vi "Initialize.vi"(8 "error in":errorcluster, 11 "Reversi in":refnum<class "Reversi.lvclass">) -> (0 "error out":errorcluster, 3 "Reversi out":refnum<class "Reversi.lvclass">)   [LabVIEW 2020, in "Reversi.lvlib" / "Reversi.lvclass"]
uses:
  Reversi.lvclass
  Space Ring.ctl
  Space Cluster.ctl
  Space Coordinates.ctl
  Reversi.lvclass/Reversi.ctl
  <vilib>/Utility/error.llb/Clear Errors.vi
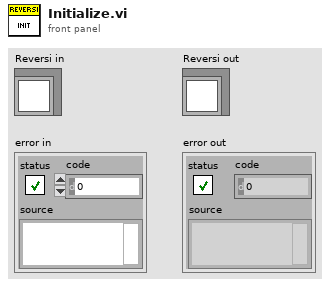
[diagram p1: front panel]
types:
  T1 = typedef "Reversi.lvlib/Reversi.lvclass/Space Cluster.ctl" = cluster{"Coordinates":T2, "Ring":T3}
  T2 = typedef "Reversi.lvlib/Reversi.lvclass/Space Coordinates.ctl" = cluster{"Row":i32, "Column":i32}
  T3 = typedef "Reversi.lvlib/Reversi.lvclass/Space Ring.ctl" = u16
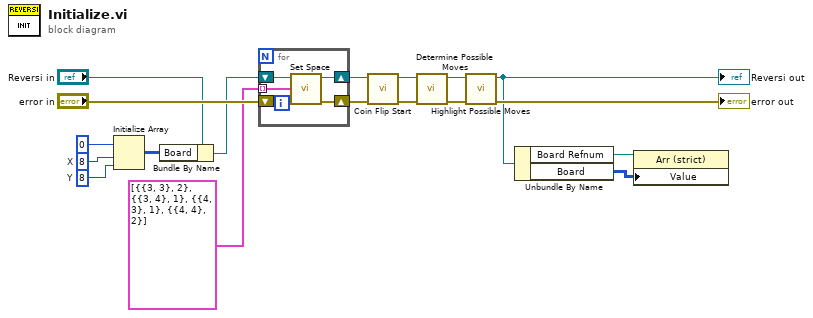
[diagram p0: block diagram]
diagram:
  w14 = 8  # Y
  w15 = 8  # X
  n1 = Initialize Array(T3 0 ("Space Ring"), w15, w14) -> (w9:T3[][])
  n2 = Bundle By Name(cluster="Reversi in", "Board"=w9) -> (w13:refnum<class "Reversi.lvclass">)
  n3 = for {
    shift-right: [w20] -> w6
    shift-left: w13 -> [w21]
    shift-right: [w22] -> w5
    shift-left: "error in" -> [w23]
    tunnel: T1[] [{"Coordinates"={"Row"=3, "Column"=3}, "Ring"=2}, {"Coordinates"={"Row"=3, "Column"=4}, "Ring"=1}, {"Coordinates"={"Row"=4, "Column"=3}, "Ring"=1}, {"Coordinates"={"Row"=4, "Column"=4}, "Ring"=2}] -> [w19] mode=indexing
    n4 = call "Set Space.vi"("error in (no error)"=w23, "Space"=w19, "Reversi in"=w21) -> ("error out"=w22:errorcluster, "Reversi out"=w20:refnum<class "Reversi.lvclass">)  [unwired: 7 in]
  }
  n5 = call "Coin Flip Start.vi"("error in (no error)"=w5, "Reversi in"=w6) -> ("error out"=w18:errorcluster, "Reversi out"=w10:refnum<class "Reversi.lvclass">)  [unwired: 8 in]
  n6 = call "Determine Possible Moves.vi"("error in (no error)"=w18, "Reversi in"=w10) -> ("error out"=w3:errorcluster, "Reversi out"=w4:refnum<class "Reversi.lvclass">)  [unwired: 8 in]
  n7 = call "Highlight Possible Moves.vi"("error in (no error)"=w3, "Reversi in"=w4) -> ("error out"=→"error out":errorcluster, "Reversi out"=w1:refnum<class "Reversi.lvclass">)  [unwired: 8 in]
  "Reversi out" <- w1
  n8 = Unbundle By Name(w1) -> ("Board Refnum"=w7:refnum<vi>, "Board"=w8:T3[][])
  n9 = property class="Arr (strict)"(reference=w7, "Value"=w8) -> ()  [unwired: 1 in, 2 out]
